vi "실습 8-1.vi"() -> ()   [LabVIEW 2014]
uses:
  System.Windows.Forms
  System.Drawing
panel:
  out "Color":u32(colorbox) caption="색"
  out "Name":string
  out "ShowDialog":i32(ring) items=["None", "OK", "Cancel", "Abort", "Retry", "Ignore", "Yes", "No"]
  out "Size":sgl
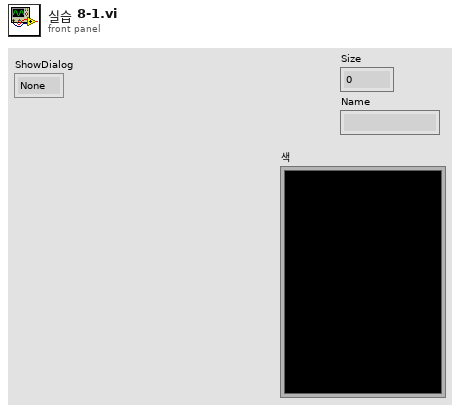
[diagram p1: front panel]
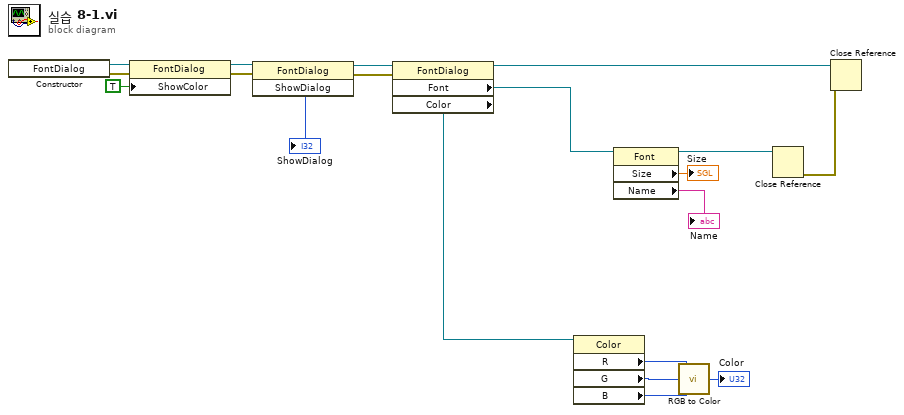
[diagram p0: block diagram]
diagram:
  n1 = constructor class="FontDialog"() -> (reference out=w12:refnum<k24>, error out=w10:errorcluster)  [unwired: 3 in, 1 out]
  n2 = property class="FontDialog"(reference=w12, error in=w10, "ShowColor"=TRUE) -> (reference out=w11:refnum<k24>, error out=w9:errorcluster)
  n3 = invoke class="FontDialog" method="ShowDialog"(reference=w11, error in=w9) -> (reference out=w19:refnum<k24>, error out=w18:errorcluster, "ShowDialog"=→"ShowDialog":i32)  [unwired: 1 in]
  n4 = property class="FontDialog"(reference=w19, error in=w18) -> (reference out=w13:refnum<k24>, "Font"=w17:refnum<k24>, "Color"=w5:refnum<k24>)  [unwired: 1 out]
  n5 = property class="Color"(reference=w5) -> ("R"=w4:u8, "G"=w3:u8, "B"=w2:u8)  [unwired: 1 in, 2 out]
  n6 = property class="Font"(reference=w17) -> (reference out=w15:refnum<k24>, "Size"=→"Size":sgl, "Name"=→"Name":string)  [unwired: 1 in, 1 out]
  n7 = call <vilib>:"RGB to Color.vi"("B"=w2, "G"=w3, "R"=w4) -> ("Color"=→"Color":u32)
  n8 = Close Reference(reference=w15) -> (error out=w14:errorcluster)  [unwired: 1 in]
  n9 = Close Reference(reference=w13, error in (no error)=w14) -> ()  [unwired: 1 out]
